vi "Shift Values.vi"(8 "error in (no error)":errorcluster, 10 "Direction":enum16{"Left", "Right", "Top", "Bottom"}(ring), 11 "Board in":refnum<class "Board.lvclass">) -> (0 "error out":errorcluster, 3 "Board out":refnum<class "Board.lvclass">)   [LabVIEW 2016, in "Board.lvclass"]
uses:
  Board.lvclass
  Block/Block.lvclass
  Board.lvclass/Board.ctl
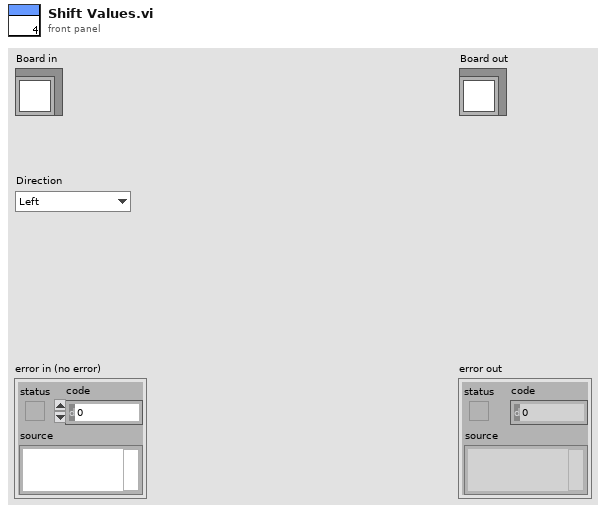
[diagram p1: front panel]
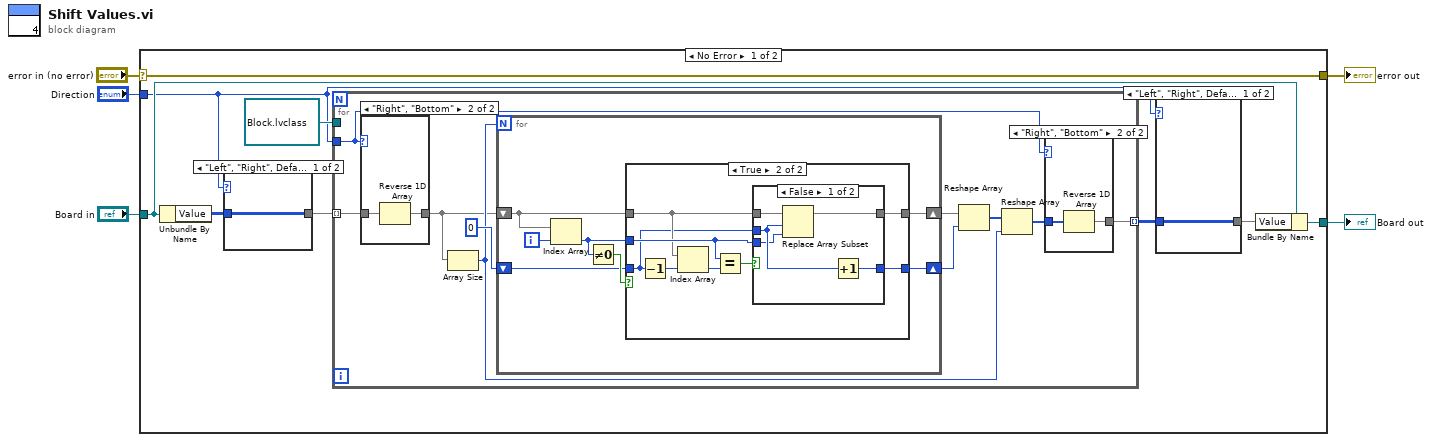
[diagram p0: block diagram]
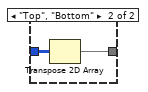
[diagram p2: hidden frame]
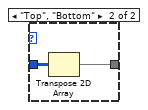
[diagram p3: hidden frame]
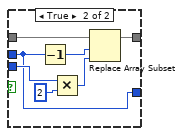
[diagram p7: hidden frame]
diagram:
  n1 = case shown="No Error" "error in (no error)" {
    selector: "error in (no error)" -> [w14 w67]
    tunnel: [w14 w67] -> w4
    tunnel: [w11 w66] -> w2
    tunnel: "Board in" -> [w12 w66]
    tunnel: "Direction" -> [w8 _]
    frame No Error {
      n2 = Unbundle By Name(w12) -> ("Value"=w10:u32[][])
      n3 = case shown="\"Left\", \"Right\", Default" w8 {
        tunnel: [w18 w19] -> w9
        tunnel: w10 -> [w18 w20]
        frame "Left", "Right", Default {
        }
        frame "Top", "Bottom" {
          n4 = Transpose 2D Array(2D array=w20) -> (transposed array=w19:u32[][])
        }
      }
      n5 = for {
        tunnel: w9 -> [w25] mode=indexing
        tunnel: refnum<data-value> refnum ("New Block") -> [_]
        tunnel: [w22] -> w7 mode=indexing
        tunnel: w8 -> [w21]
        n6 = case shown="\"Right\", \"Bottom\"" w21 {
          tunnel: w25 -> [w34 w36]
          tunnel: [w34 w35] -> w24
          frame "Left", "Top", Default {
          }
          frame "Right", "Bottom" {
            n7 = Reverse 1D Array(array=w36) -> (reversed array=w35:u32[])
          }
        }
        n8 = Array Size(array=w24) -> (size(s)=w27:i32)
        n9 = for {
          N: w27 -> [_]
          shift-right: [w40] -> w30
          shift-left: w24 -> [w38]
          shift-right: [w39] -> w26
          shift-left: 0 -> [w37]
          i -> [w41]
          n10 = Index Array(array=w38, index=w41) -> (element=w42:u32)
          n11 = Not Equal To 0?(x=w42) -> (x != 0?=w43:bool)
          n12 = case shown="True" w43 {
            tunnel: w38 -> [w45 w48]
            tunnel: w37 -> [w44 w47]
            tunnel: [w44 w51] -> w39
            tunnel: [w45 w50] -> w40
            tunnel: w42 -> [_ w52]
            frame False {
            }
            frame True {
              n13 = Decrement(x=w47) -> (x-1=w49:i32)
              n14 = Index Array(array=w48, index=w49) -> (element=w46:u32)
              n15 = Equal?(x=w52, y=w46) -> (x = y?=w53:bool)
              n16 = case shown="False" w53 {
                tunnel: w52 -> [w55 w65]
                tunnel: w47 -> [w56 w61]
                tunnel: [w58 w61] -> w51
                tunnel: w48 -> [w57 w63]
                tunnel: [w54 w59] -> w50
                frame False {
                  n17 = Replace Array Subset(array=w57, new element=w55, index=w56) -> (w54:u32[])
                  n18 = Increment(x=w56) -> (x+1=w58:i32)
                }
                frame True {
                  n19 = Decrement(x=w61) -> (x-1=w60:i32)
                  n20 = Multiply(x=w65, y=u32 2) -> (x*y=w62:u32)
                  n21 = Replace Array Subset(array=w63, new element=w62, index=w60) -> (w59:u32[])
                }
              }
            }
          }
        }
        n22 = Reshape Array(w30, w26) -> (w28:u32[])
        n23 = Reshape Array(w28, w27) -> (w23:u32[])
        n24 = case shown="\"Right\", \"Bottom\"" w21 {
          tunnel: w23 -> [w31 w33]
          tunnel: [w31 w32] -> w22
          frame "Left", "Top", Default {
          }
          frame "Right", "Bottom" {
            n25 = Reverse 1D Array(array=w33) -> (reversed array=w32:u32[])
          }
        }
      }
      n26 = case shown="\"Left\", \"Right\", Default" w8 {
        tunnel: [w15 w16] -> w6
        tunnel: w7 -> [w15 w17]
        frame "Left", "Right", Default {
        }
        frame "Top", "Bottom" {
          n27 = Transpose 2D Array(2D array=w17) -> (transposed array=w16:u32[][])
        }
      }
      n28 = Bundle By Name(cluster=w12, "Value"=w6) -> (w11:refnum<class "Board.lvclass">)
    }
    frame Error {
    }
  }
  "error out" <- w4
  "Board out" <- w2
